vi "IAmGLF-CreateDVR.vi"(8 "error in (no error)":errorcluster, 11 "Window in":refnum<class "Window.lvclass">) -> (0 "error out":errorcluster, 3 "Window out":refnum<class "Window.lvclass">)   [LabVIEW 2024, in "GLF.lvlib" / "Window.lvclass"]
doc: "<B>Summary</B>\nTo create the class DVR in an standalone process."
uses:
  Window.lvclass
  Window.lvclass/Window.ctl
  DVR--cluster.ctl
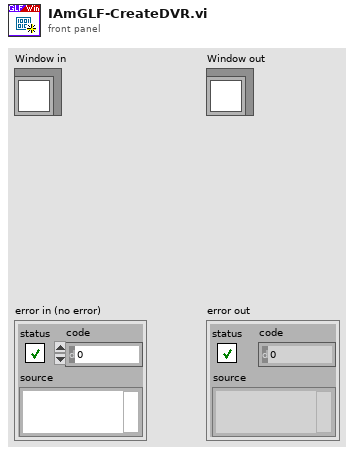
[diagram p1: front panel]
types:
  T1 = typedef "GLF.lvlib/Window.lvclass/DVR--cluster.ctl" = cluster{"foo":dbl}
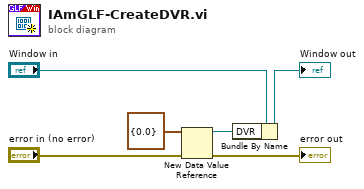
[diagram p0: block diagram]
diagram:
  n1 = New Data Value Reference(data value=T1 {"foo"=0.0} ("DVR"), error in="error in (no error)") -> (data value reference=w3:refnum<data-value>, error out=→"error out":errorcluster)
  n2 = Bundle By Name(cluster="Window in", "DVR"=w3) -> (→"Window out":refnum<class "Window.lvclass">)
